vi "PLC Array Byte Stream to Data String.vi"(8 "error in (no error)":errorcluster, 9 "Array Type Descriptor":T1, 10 "Byte Stream":u8[](array[numeric]), 11 "TwinCAT ADS in":refnum<class "TwinCAT ADS.lvclass">) -> (0 "error out":errorcluster, 1 "Data String":string, 2 "Type Descriptor":i16[](array[numeric]), 3 "TwinCAT ADS out":refnum<class "TwinCAT ADS.lvclass">)   [LabVIEW 2018, in "TwinCAT ADS.lvclass"]
uses:
  TwinCAT ADS.lvclass
  Controls/PLC Array Type Descriptor.ctl
  Controls/PLC Type.ctl
  Controls/PLC Sub-Item Type Descriptor.ctl
  PLC Primitive Byte Stream to Data String.vi/dd5e40b3-f89d-44d0-b911-1f2dc1f1e391.vi
  PLC Primitive Byte Stream to Data String.vi/9a8c356b-cf55-4838-9201-0532b80217b2.vi
  PLC Primitive Byte Stream to Data String.vi/06482052-d1f9-4f29-aca9-908031c6a69f.vi
  PLC Primitive Byte Stream to Data String.vi/b9242781-96b0-446e-9150-452b1084ed54.vi
  PLC Primitive Byte Stream to Data String.vi/5fbe6976-0b86-40a2-b7b6-3748894f0071.vi
  PLC Primitive Byte Stream to Data String.vi/c4de1741-fffd-4fed-ba25-d7b4acbf0555.vi
  PLC Primitive Byte Stream to Data String.vi/20356124-05d2-4a04-a5d1-e69adc4c58c2.vi
  PLC Primitive Byte Stream to Data String.vi/67ddb754-0fbe-43d9-9e61-34d6659124ef.vi
  PLC Primitive Byte Stream to Data String.vi/e3d41cb3-d20e-45e9-8252-e41884a8f4d0.vi
  PLC Primitive Byte Stream to Data String.vi/46ba2a54-cc07-4222-9a0e-bd972edfcef0.vi
  PLC Primitive Byte Stream to Data String.vi/6b416cf7-30dc-48a3-9278-9d800f443678.vi
  PLC Primitive Byte Stream to Data String.vi/5857d013-9824-4299-a2d7-53efdc0d26c5.vi
  PLC Primitive Byte Stream to Data String.vi/006b0e7e-7e80-41f3-be4e-1f3da8479fae.vi
  PLC Primitive Byte Stream to Data String.vi/28d9c90b-5f2a-4c58-95e2-5fc46303b0fd.vi
  PLC Primitive Byte Stream to Data String.vi/99b7bc4a-962e-4818-aa5d-444f23f83b11.vi
  PLC Primitive Byte Stream to Data String.vi/8b7c42c8-9170-4542-8f35-15cbeddc22cb.vi
  PLC Primitive Byte Stream to Data String.vi/65a091fa-0bd2-4a35-ae2b-3fa5e90d1994.vi
  PLC Primitive Byte Stream to Data String.vi/4b7d3a7d-7f1b-46f0-9357-48cb72148c56.vi
  PLC Primitive Byte Stream to Data String.vi/b431183c-2ad5-4c6d-9bfa-a53b18913682.vi
  PLC Primitive Byte Stream to Data String.vi/30c6c28a-53c3-4e33-80b1-b22f521e1f67.vi
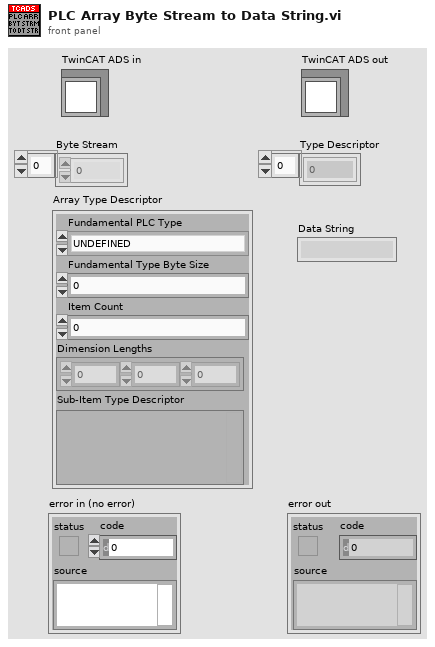
[diagram p1: front panel]
types:
  T1 = typedef "TwinCAT ADS.lvclass/PLC Array Type Descriptor.ctl" = cluster{"Fundamental PLC Type":T2, "Fundamental Type Byte Size":i32, "Item Count":i32, "Dimension Lengths":i32[], "Sub-Item Type Descriptor":variant}
  T2 = typedef "TwinCAT ADS.lvclass/PLC Type.ctl" = enum16{"UNDEFINED", "INT", "DINT", "REAL", "LREAL", "SINT", "BYTE", "UINT", "UDINT", "LINT", "ULINT", "STRING", "WSTRING", "BOOL", "TIME", "LTIME", "DATE", "DT", "TOD", "ARRAY", "JAGGED ARRAY", "STRUCT", "FUNCTION BLOCK", "UNION", "POINTER", "USER DEFINED"}
  T3 = typedef "TwinCAT ADS.lvclass/PLC Sub-Item Type Descriptor.ctl" = cluster{"PLC Type":T2, "Offset":i32, "Byte Size":i32, "[Sub-Item/Array Type Descriptor]":variant[]}
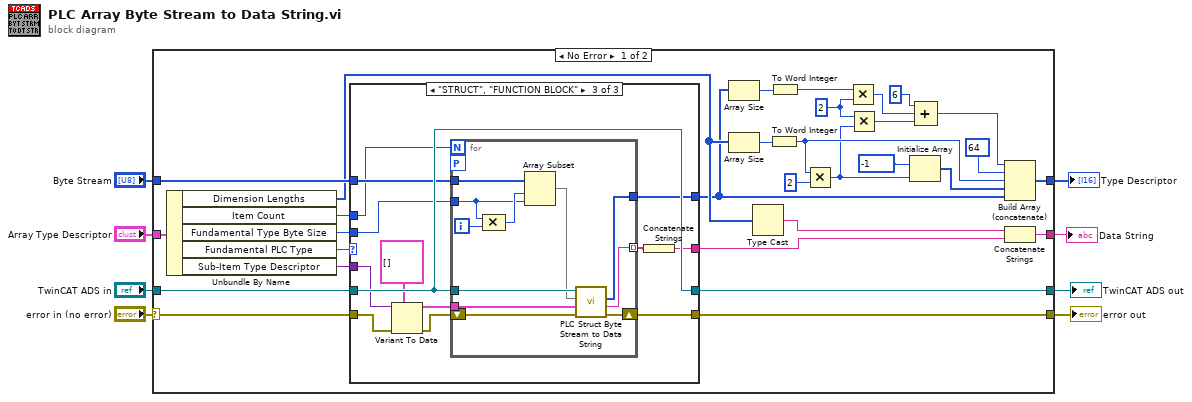
[diagram p0: block diagram]
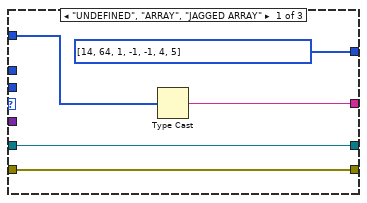
[diagram p2: hidden frame]
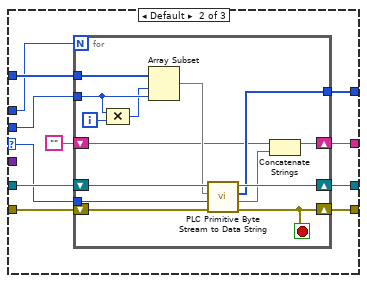
[diagram p3: hidden frame]
diagram:
  n1 = case shown="No Error" "error in (no error)" {
    selector: "error in (no error)" -> [w30 w93]
    tunnel: "TwinCAT ADS in" -> [w38 w94]
    tunnel: "Byte Stream" -> [w37 _]
    tunnel: [w9 w93] -> w6
    tunnel: [w36 w94] -> w5
    tunnel: "Array Type Descriptor" -> [w35 _]
    tunnel: [w28 _] -> w1
    tunnel: [w26 _] -> w2
    frame No Error {
      w15 = i16 2 ("y")
      n2 = Unbundle By Name(w35) -> ("Dimension Lengths"=w24:i32[], "Item Count"=w33:i32, "Fundamental Type Byte Size"=w31:i32, "Fundamental PLC Type"=w32:T2, "Sub-Item Type Descriptor"=w34:variant)
      n3 = case shown="\"STRUCT\", \"FUNCTION BLOCK\"" w32 {
        selector: w32 -> [_ w50 _]
        tunnel: w30 -> [w42 w54 w76]
        tunnel: w38 -> [w43 w53 w81]
        tunnel: w37 -> [w41 w48 w79]
        tunnel: [w42 w52 w80] -> w9
        tunnel: [w43 w51 w81] -> w36
        tunnel: w34 -> [_ _ w75]
        tunnel: w33 -> [_ w47 w78]
        tunnel: w31 -> [_ w49 w77]
        tunnel: [w40 w45 w69] -> w27
        tunnel: [i16[] [14, 64, 1, -1, -1, 4, 5] ("Type Descriptor") w44 w71] -> w19
        frame "UNDEFINED", "ARRAY", "JAGGED ARRAY" {
          n4 = Type Cast(x=w41) -> (*(type *) &x=w40:string)  [unwired: 1 in]
        }
        frame Default {
          n5 = for {
            N: w47 -> [_]
            shift-right: [w60] -> w51
            shift-left: w53 -> [w64]
            tunnel: w50 -> [w62]
            tunnel: w49 -> [w66]
            shift-right: [w59] -> w52
            shift-left: w54 -> [w63]
            tunnel: w48 -> [w68]
            shift-right: [w57] -> w45
            shift-left: "" -> [w55]
            tunnel: [w56] -> w44
            i -> [w67]
            stop <- w59 stop-if-true
            n6 = Compound Arithmetic op=MULTIPLY(w66, w67) -> (w65:i32)
            n7 = Array Subset(array=w68, index=w65, length=w66) -> (w61:u8[])
            n8 = call "PLC Primitive Byte Stream to Data String.vi"("error in (no error)"=w63, "PLC Type"=w62, "Byte Stream"=w61, "TwinCAT ADS in"=w64) -> ("error out"=w59:errorcluster, "Data String"=w58:string, "Type Descriptor"=w56:i16[], "TwinCAT ADS out"=w60:refnum<class "TwinCAT ADS.lvclass">)  [unwired: 4 in]
            n9 = Concatenate Strings(w55, w58) -> (w57:string)
          }
        }
        frame "STRUCT", "FUNCTION BLOCK" {
          n10 = Variant To Data(error in=w76, type=T3[] [] ("[Sub-Item Type Information]"), Variant=w75) -> (data=w72:T3[], error out=w74:errorcluster)
          n11 = for {
            N: w78 -> [_]
            tunnel: w77 -> [w89]
            tunnel: w72 -> [w86]
            shift-right: [w82] -> w80
            shift-left: w74 -> [w87]
            tunnel: w79 -> [w91]
            workers-P: _ -> [_]
            tunnel: w81 -> [w88]
            tunnel: [w84] -> w71
            tunnel: [w83] -> w70 mode=indexing
            i -> [w90]
            n12 = Compound Arithmetic op=MULTIPLY(w89, w90) -> (w92:i32)
            n13 = Array Subset(array=w91, index=w92, length=w89) -> (w85:u8[])
            n14 = call "PLC Struct Byte Stream to Data String.vi"("error in (no error)"=w87, "[Sub-Item Type Information]"=w86, "Byte Stream"=w85, "TwinCAT ADS in"=w88) -> ("error out"=w82:errorcluster, "Data String"=w83:string, "Type Descriptor"=w84:i16[])  [unwired: 4 in, 1 out]
          }
          n15 = Concatenate Strings(w70) -> (w69:string)
        }
      }
      n16 = Array Size(array=w19) -> (size(s)=w18:i32)
      n17 = Array Size(array=w24) -> (size(s)=w29:i32)
      n18 = Type Cast(x=w24) -> (*(type *) &x=w25:string)  [unwired: 1 in]
      n19 = To Word Integer(number=w29) -> (16bit integer=w22:i16)
      n20 = To Word Integer(number=w18) -> (16bit integer=w17:i16)
      n21 = Multiply(x=w22, y=i16 2) -> (x*y=w16:i16)
      n22 = Multiply(x=w17, y=w15) -> (x*y=w14:i16)
      n23 = Multiply(x=w15, y=w16) -> (x*y=w13:i16)
      n24 = Initialize Array(i16 -1, w16) -> (w20:i16[])
      n25 = Compound Arithmetic op=ADD(i16 6 ("y"), w14, w13) -> (w10:i16)
      n26 = Build Array (concatenate)(w10, i16 64, w22, w20, w19) -> (w28:i16[])
      n27 = Concatenate Strings(w25, w27) -> (w26:string)
    }
    frame Error {
    }
  }
  "error out" <- w6
  "TwinCAT ADS out" <- w5
  "Type Descriptor" <- w1
  "Data String" <- w2
